vi "svl_Max-Min Resampled Level with IC.vi"(6 "initial min level":dbl format="%.2f", 7 "initial max level":dbl format="%.2f", 8 "error in (no error)":errorcluster, 9 "processing state":T2(ring), 11 "even angle signal":T1 {"even angle signal" format="%.2f"; "dr" format="%.2f"; "r0" format="%.2f"}) -> (0 "error out":errorcluster, 2 "max-min level":dbl format="%.2f", 4 "final min level":dbl format="%.2f", 5 "final max level":dbl format="%.2f")   [LabVIEW 2017]
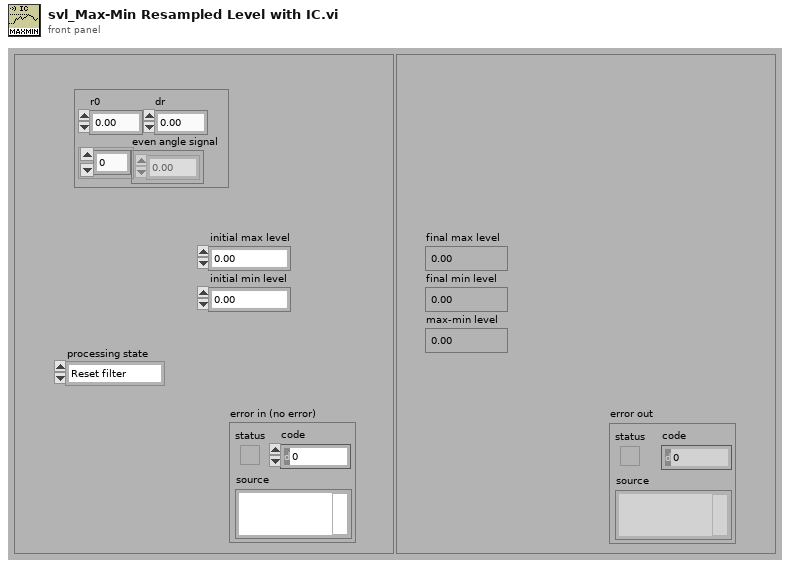
[diagram p1: front panel]
types:
  T1 = cluster{"r0":dbl, "dr":dbl, "even angle signal":dbl[]}
  T2 = enum16{"Reset filter", "Restart averaging", "Continue processing"}
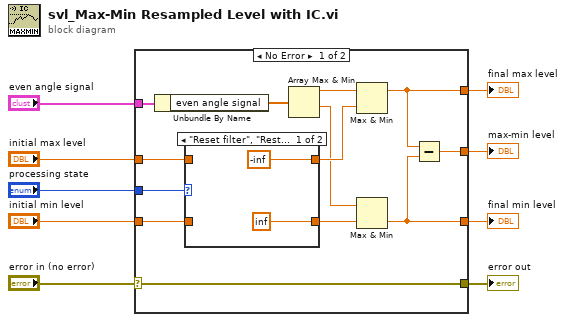
[diagram p0: block diagram]
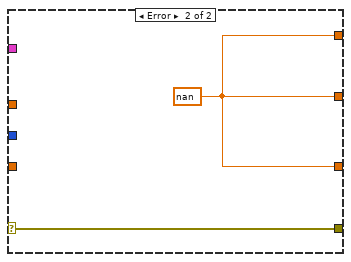
[diagram p3: hidden frame]
diagram:
  n1 = case shown="No Error" "error in (no error)" {
    selector: "error in (no error)" -> [w22 w28]
    tunnel: [w22 w28] -> w7
    tunnel: "even angle signal" -> [w11 _]
    tunnel: "processing state" -> [w21 _]
    tunnel: "initial max level" -> [w18 _]
    tunnel: [w14 w27] -> w9
    tunnel: "initial min level" -> [w19 _]
    tunnel: [w13 w27] -> w2
    tunnel: [w12 w27] -> w1
    frame No Error {
      n2 = Unbundle By Name(w11) -> ("even angle signal"=w10:dbl[])
      n3 = case shown="\"Reset filter\", \"Restart averaging\", Default" w21 {
        tunnel: w18 -> [_ w26]
        tunnel: [-inf ("t") w26] -> w17
        tunnel: w19 -> [_ w25]
        tunnel: [inf ("t") w25] -> w15
        frame "Reset filter", "Restart averaging", Default {
        }
        frame "Continue processing" {
        }
      }
      n4 = Array Max & Min(array=w10) -> (max value=w20:dbl, min value=w16:dbl)  [unwired: 2 out]
      n5 = Max & Min(x=w20, y=w17) -> (max(x,y)=w14:dbl)  [unwired: 1 out]
      n6 = Max & Min(x=w16, y=w15) -> (min(x,y)=w13:dbl)  [unwired: 1 out]
      n7 = Subtract(x=w14, y=w13) -> (x-y=w12:dbl)
    }
    frame Error {
      w27 = nan ("soundLevel")
    }
  }
  "final max level" <- w9
  "error out" <- w7
  "final min level" <- w2
  "max-min level" <- w1
